vi "Rule Filter.vi"(1 "WiringRules[]":T1(array[ring])) -> (0 "wiring rules":T1(array[ring]))   [LabVIEW 2016]
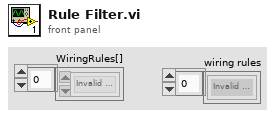
[diagram p1: front panel]
types:
  T1 = enum16{"Invalid Wire Rule", "Required", "Recommended", "Optional", "Dynamic Dispatch"}[]
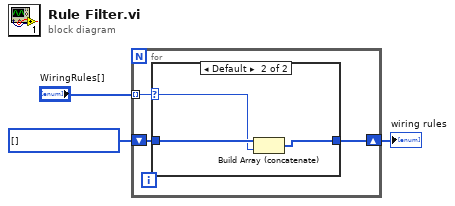
[diagram p0: block diagram]
diagram:
  w3 = T1 [] items=["Invalid Wire Rule", "Required", "Recommended", "Optional", "Dynamic Dispatch"]
  n1 = for {
    tunnel: "WiringRules[]" -> [w6] mode=indexing
    shift-right: [w4] -> w1
    shift-left: w3 -> [w5]
    n2 = case shown="Default" w6 {
      selector: w6 -> [_ w9]
      tunnel: w5 -> [w7 w10]
      tunnel: [w7 w8] -> w4
      frame "Invalid Wire Rule" {
      }
      frame Default {
        n3 = Build Array (concatenate)(w10, w9) -> (w8:T1)
      }
    }
  }
  "wiring rules" <- w1
